vi "S2C_VLFT10_Proc_SetSerialNumber.vi"(8 "Error In":errorcluster, 11 "SN In":string) -> (0 "Error Out":errorcluster, 3 "Result":string)   [LabVIEW 2015]
uses:
  Fornax/VIs/PolyDriver/Typedefs/BoardId.ctl
  Fornax/VIs/PolyDriver/Typedefs/BoardIdDataSet.ctl
  Fornax/VIs/PolyDriver/Typedefs/BoardIdCommand.ctl
  Fornax/VIs/PolyDriver/Typedefs/SystemConfigurationCommand.ctl
  Fornax/VIs/PolyDriver/S2C_FORNAX_Poly_BoardIdCommand.vi
  Fornax/VIs/PolyDriver/S2C_FORNAX_Poly_SystemConfigurationCommand.vi
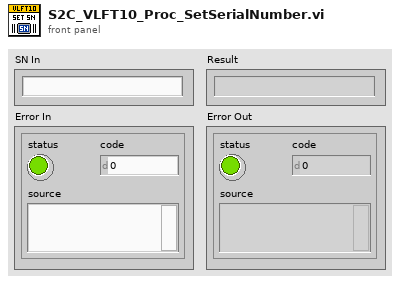
[diagram p1: front panel]
types:
  T1 = typedef "BoardId.ctl" = i16
  T2 = typedef "BoardIdDataSet.ctl" = i16
  T3 = typedef "BoardIdCommand.ctl" = i16
  T4 = cluster{"Partition":string, "Message":string, "M_BoardId":T1, "M_BoardIdDataSet":T2, "M_Command":T3, "M_Value":string}
  T5 = cluster{"Driver":string, "Command":string, "Return":string, "Parameters":string, "Timeout":dbl}
  T6 = typedef "SystemConfigurationCommand.ctl" = i16
  T7 = cluster{"Partition":string, "Message":string, "M_Command":T6, "M_ConfigurationData":string}
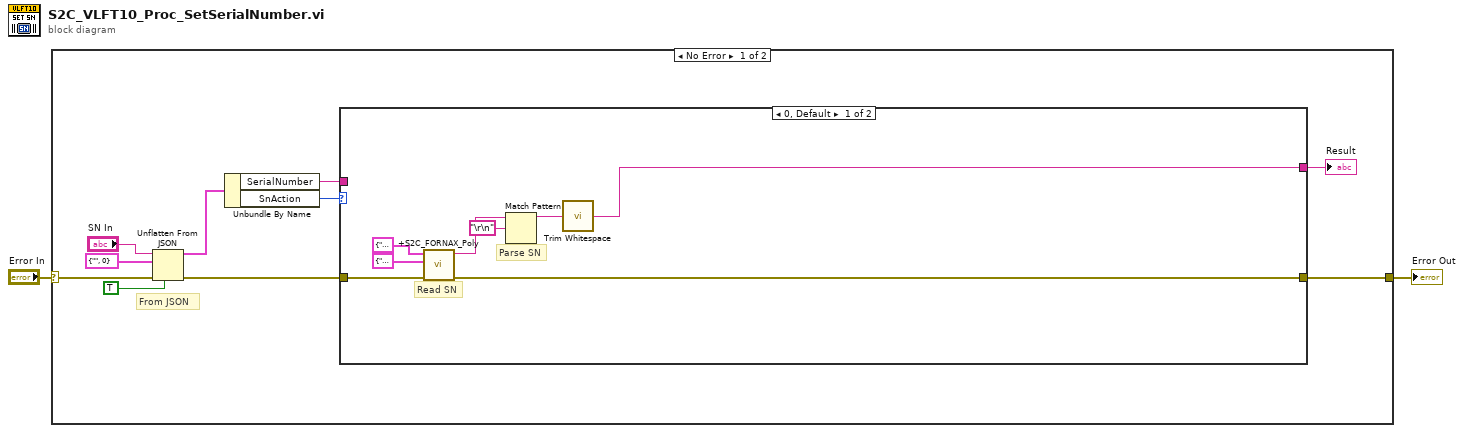
[diagram p0: block diagram]
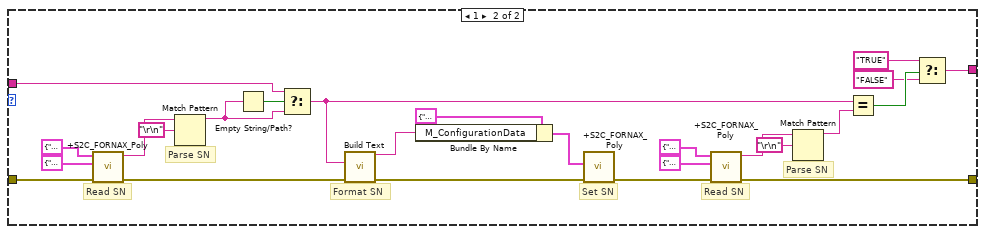
[diagram p2: hidden frame]
diagram:
  n1 = case shown="No Error" "Error In" {
    selector: "Error In" -> [w12 w46]
    tunnel: [w6 w46] -> w1
    frame No Error {
      # "From JSON"
      n2 = Unflatten From JSON(JSON string="SN In", type and defaults=cluster{"SerialNumber":string, "SnAction":u16} {"SerialNumber"="", "SnAction"=0}, default null elements? (F)=TRUE, error in (no error)=w12) -> (value=w8:cluster{"SerialNumber":string, "SnAction":u16}, error out=w11:errorcluster)  [unwired: 3 in]
      n3 = Unbundle By Name(w8) -> ("SerialNumber"=w7:string, "SnAction"=w4:u16)
      n4 = case shown="0, Default" w4 {
        tunnel: w11 -> [w16 w31]
        tunnel: w7 -> [_ w29]
        tunnel: [w15 w27] -> w6
        tunnel: [w13 w21] -> w3
        frame 0, Default {
          # "Parse SN"
          # "Read SN"
          n5 = call-poly "+S2C_FORNAX_Poly.vi"("Error In"=w16, "BoardIdCommand"=T4 {"Partition"="Default", "Message"="BoardIdCommand", "M_BoardId"=1, "M_BoardIdDataSet"=2, "M_Command"=2, "M_Value"=""}, "Settings"=T5 {"Driver"="Fornax", "Command"="BoardIdCommand", "Return"="M_Value", "Parameters"="", "Timeout"=10.0}) -> ("Error Out"=w15:errorcluster, "Response"=w18:string)  [unwired: 7 in]
          n6 = Match Pattern(string=w18, regular expression="\r\n") -> (before substring=w14:string)  [unwired: 1 in, 3 out]
          n7 = call <vilib>:"Trim Whitespace.vi"("string"=w14) -> ("trimmed string"=w13:string)  [unwired: 1 in]
        }
        frame 1 {
          # "Parse SN"
          # "Read SN"
          # "Set SN"
          # "Format SN"
          # "Parse SN"
          # "Read SN"
          n8 = call-poly "+S2C_FORNAX_Poly.vi"("Error In"=w31, "BoardIdCommand"=T4 {"Partition"="Default", "Message"="BoardIdCommand", "M_BoardId"=1, "M_BoardIdDataSet"=2, "M_Command"=2, "M_Value"=""}, "Settings"=T5 {"Driver"="Fornax", "Command"="BoardIdCommand", "Return"="M_Value", "Parameters"="", "Timeout"=10.0}) -> ("Error Out"=w41:errorcluster, "Response"=w43:string)  [unwired: 7 in]
          n9 = Match Pattern(string=w43, regular expression="\r\n") -> (before substring=w28:string)  [unwired: 1 in, 3 out]
          n10 = Empty String/Path?(string/path=w28) -> (empty?=w30:bool)
          n11 = Select(t=w29, s=w30, f=w28) -> (s? t:f=w26:string)
          n12 = call "Build Text"("SN"=w26, "error in (no error)"=w41) -> ("Result"=w37:string, "error out"=w40:errorcluster)  [unwired: 12 in]
          n13 = Bundle By Name(cluster=T7 {"Partition"="Default", "Message"="SystemConfigurationCommand", "M_Command"=7, "M_ConfigurationData"=""} ("SystemConfigurationCommand"), "M_ConfigurationData"=w37) -> (w38:T7)
          n14 = call-poly "+S2C_FORNAX_Poly.vi"("Error In"=w40, "SystemConfigurationCommand"=w38) -> ("Error Out"=w32:errorcluster)  [unwired: 8 in, 1 out]
          n15 = call-poly "+S2C_FORNAX_Poly.vi"("Error In"=w32, "BoardIdCommand"=T4 {"Partition"="Default", "Message"="BoardIdCommand", "M_BoardId"=1, "M_BoardIdDataSet"=2, "M_Command"=2, "M_Value"=""}, "Settings"=T5 {"Driver"="Fornax", "Command"="BoardIdCommand", "Return"="M_Value", "Parameters"="", "Timeout"=10.0}) -> ("Error Out"=w27:errorcluster, "Response"=w35:string)  [unwired: 7 in]
          n16 = Match Pattern(string=w35, regular expression="\r\n") -> (before substring=w25:string)  [unwired: 1 in, 3 out]
          n17 = Equal?(x=w26, y=w25) -> (x = y?=w24:bool)
          n18 = Select(t="TRUE", s=w24, f="FALSE") -> (s? t:f=w21:string)
        }
      }
      "Result" <- w3
    }
    frame Error {
    }
  }
  "Error Out" <- w1
